vi "Bundle.vi"(8 "error in (no error)":errorcluster, 9 "Connection Type":T1=enum."SwitchBlock Device", 10 "Alias":string, 11 "Instrument in":refnum<class "Instrument Driver.lvclass">) -> (0 "error out":errorcluster, 3 "Instrument out":refnum<class "Instrument Driver.lvclass">)   [LabVIEW 2020, in "Instrument Driver.lvlib" / "Instrument Driver.lvclass"]
doc: "Write the Alias and Connection Type to the Instrument."
uses:
  Instrument Driver.lvclass
  Controls/Ctl_ConnectionType.ctl
  Instrument Driver.lvclass/Instrument Driver.ctl
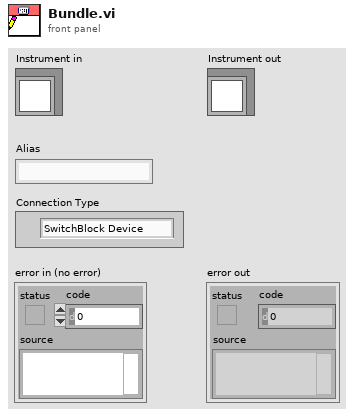
[diagram p1: front panel]
types:
  T1 = typedef "Instrument Driver.lvlib/Instrument Driver.lvclass/Ctl_ConnectionType.ctl" = enum16{"BuiltIn/System", "PXI/PCI", "USB", "GPIB", "VXI", "Serial", "TCP/IP", "cRIO", "SCXI", "cDAQ", "SwitchBlock", "SCC", "FireWire", "Accessory", "CAN", "SwitchBlock Device"}
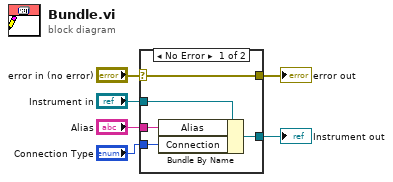
[diagram p0: block diagram]
diagram:
  n1 = case shown="No Error" "error in (no error)" {
    selector: "error in (no error)" -> [w11 w12]
    tunnel: [w11 w12] -> w5
    tunnel: [w9 w13] -> w3
    tunnel: "Instrument in" -> [w10 w13]
    tunnel: "Alias" -> [w8 _]
    tunnel: "Connection Type" -> [w7 _]
    frame No Error {
      n2 = Bundle By Name(cluster=w10, "Alias"=w8, "Connection"=w7) -> (w9:refnum<class "Instrument Driver.lvclass">)
    }
    frame Error {
    }
  }
  "error out" <- w5
  "Instrument out" <- w3
